vi "Caption Set Avg Fuel.vi"(0 "Reference Cluster":T1, 1 "Slave ID":dbl=128.0 format="%#_13g") -> ()   [LabVIEW 2017, in "GUI.lvlib"]
uses:
  GUI.lvlib
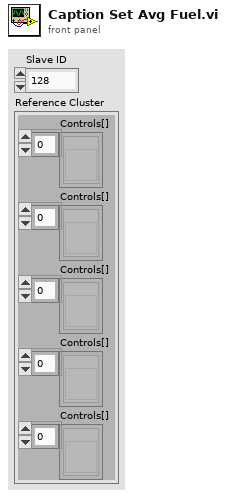
[diagram p1: front panel]
types:
  T1 = cluster{"Controls[]":refnum<vi>[], "Controls[]":refnum<vi>[], "Controls[]":refnum<vi>[], "Controls[]":refnum<vi>[], "Controls[]":refnum<vi>[]}
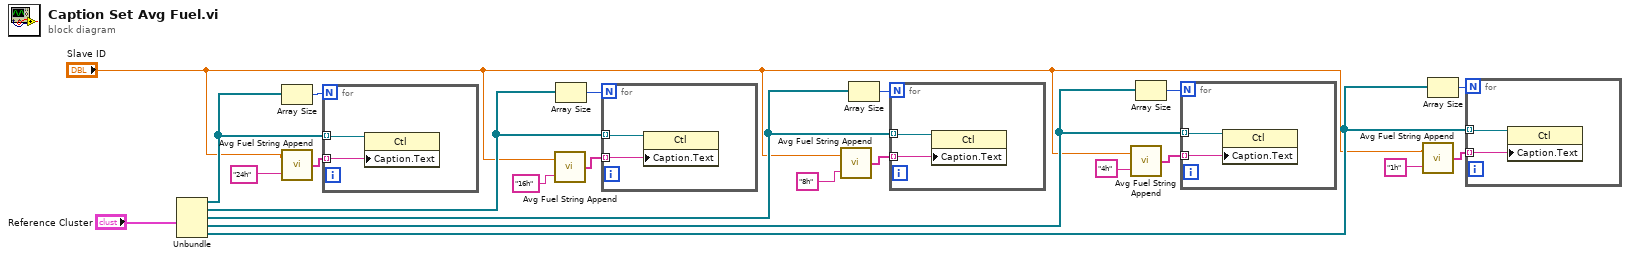
[diagram p0: block diagram]
diagram:
  n1 = Unbundle("Reference Cluster") -> ("Controls[]"=w22:refnum<vi>[], "Controls[]"=w19:refnum<vi>[], "Controls[]"=w17:refnum<vi>[], "Controls[]"=w15:refnum<vi>[], "Controls[]"=w13:refnum<vi>[])
  n2 = Array Size(array=w22) -> (size(s)=w21:i32)
  n3 = call "Avg Fuel String Append.vi"("Append String"="24h", "Slave ID"="Slave ID") -> ("Avg captions"=w8:string[])
  n4 = for {
    N: w21 -> [_]
    tunnel: w22 -> [w24] mode=indexing
    tunnel: w8 -> [w23] mode=indexing
    n5 = property class="Ctl"(reference=w24, "Caption.Text"=w23) -> ()  [unwired: 1 in, 2 out]
  }
  n6 = call "Avg Fuel String Append.vi"("Append String"="16h", "Slave ID"="Slave ID") -> ("Avg captions"=w10:string[])
  n7 = Array Size(array=w19) -> (size(s)=w20:i32)
  n8 = for {
    N: w20 -> [_]
    tunnel: w19 -> [w26] mode=indexing
    tunnel: w10 -> [w25] mode=indexing
    n9 = property class="Ctl"(reference=w26, "Caption.Text"=w25) -> ()  [unwired: 1 in, 2 out]
  }
  n10 = call "Avg Fuel String Append.vi"("Append String"="8h", "Slave ID"="Slave ID") -> ("Avg captions"=w7:string[])
  n11 = Array Size(array=w17) -> (size(s)=w18:i32)
  n12 = for {
    N: w18 -> [_]
    tunnel: w17 -> [w28] mode=indexing
    tunnel: w7 -> [w27] mode=indexing
    n13 = property class="Ctl"(reference=w28, "Caption.Text"=w27) -> ()  [unwired: 1 in, 2 out]
  }
  n14 = call "Avg Fuel String Append.vi"("Append String"="4h", "Slave ID"="Slave ID") -> ("Avg captions"=w5:string[])
  n15 = Array Size(array=w15) -> (size(s)=w16:i32)
  n16 = for {
    N: w16 -> [_]
    tunnel: w15 -> [w30] mode=indexing
    tunnel: w5 -> [w29] mode=indexing
    n17 = property class="Ctl"(reference=w30, "Caption.Text"=w29) -> ()  [unwired: 1 in, 2 out]
  }
  n18 = call "Avg Fuel String Append.vi"("Append String"="1h", "Slave ID"="Slave ID") -> ("Avg captions"=w3:string[])
  n19 = Array Size(array=w13) -> (size(s)=w14:i32)
  n20 = for {
    N: w14 -> [_]
    tunnel: w13 -> [w32] mode=indexing
    tunnel: w3 -> [w31] mode=indexing
    n21 = property class="Ctl"(reference=w32, "Caption.Text"=w31) -> ()  [unwired: 1 in, 2 out]
  }
